vi "dsdll_enumerate_devices.vi"(5 "capture devices ring ref":refnum<vi>, 7 "output devices ring ref":refnum<vi>, 8 "error in":errorcluster, 11 "dsdll instance in":T2={"dsdll path"=path "E:/LVprog/DirectSoundDLL/dsdll.dll", "dsdll handle"=[], "output devices"=[], "capture devices"=[]}) -> (0 "error out":errorcluster, 1 "capture device list":T1[](array[typedef]), 2 "output device list":T1[](array[typedef]), 3 "dsdll instance out":T2)   [LabVIEW 2020, in "dsdll.lvlib"]
doc: "Call this to enumerate output and capture devices. Must be called before opening the audio devices.\n\nThe VI returns lists of output and capture devices and optionally it fills ring buffers with the names of the found devices.\n\nIMPORTANT: The lists of the enumerated devices are also stored in the DSDLL instance handle so don't discard it because it will be later used to open the devices!"
uses:
  dsdll.lvlib
  dsdll_instance.ctl
  dsdll_device_record.ctl
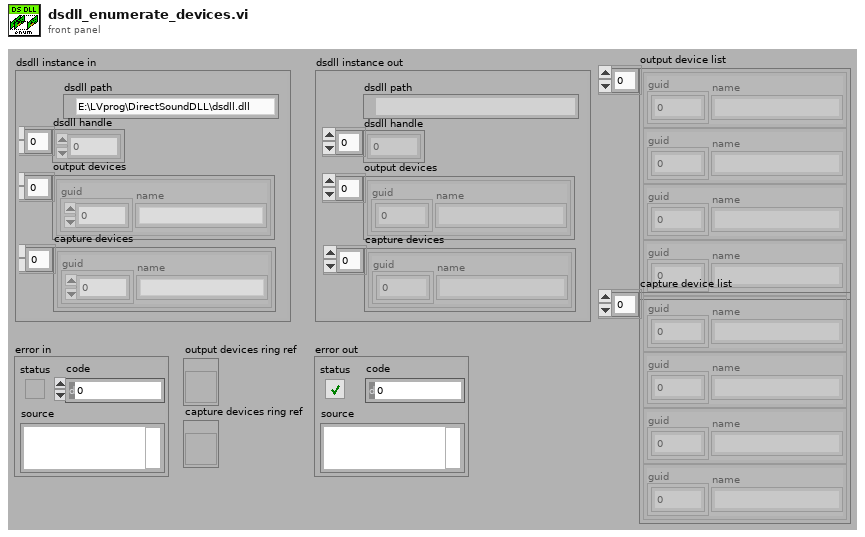
[diagram p1: front panel]
types:
  T1 = typedef "dsdll.lvlib/dsdll_device_record.ctl" = cluster{"guid":u8[], "name":string}
  T2 = typedef "dsdll.lvlib/dsdll_instance.ctl" = cluster{"dsdll path":path, "dsdll handle":u8[], "output devices":T1[], "capture devices":T1[]}
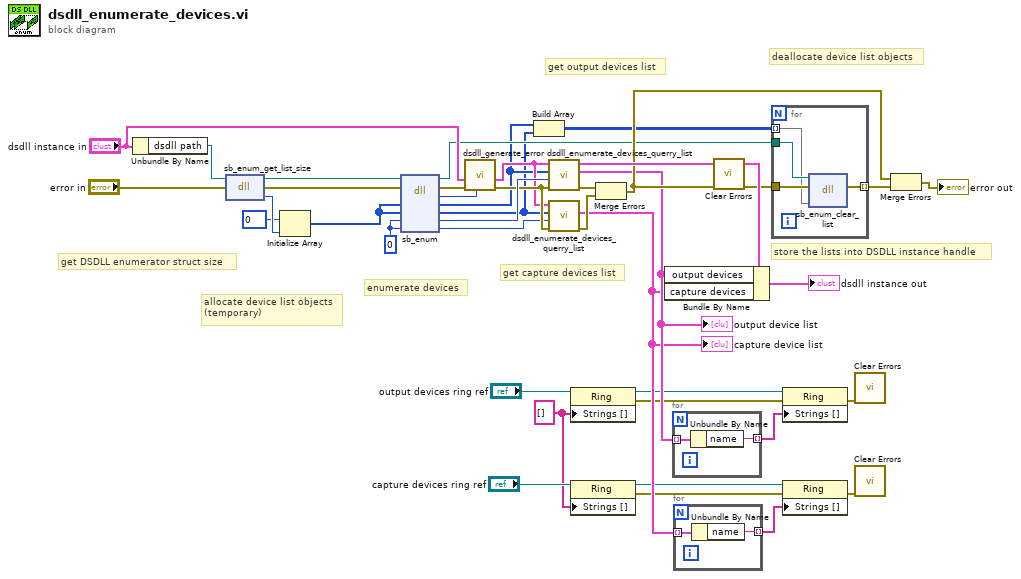
[diagram p0: block diagram]
diagram:
  w1 = string[] [] ("Strings []")
  w31 = 0
  # "deallocate device list objects"
  # "allocate device list objects\n(temporary)"
  # "store the lists into DSDLL instance handle"
  # "get capture devices list"
  # "get output devices list"
  # "enumerate devices"
  # "get DSDLL enumerator struct size"
  n1 = Unbundle By Name("dsdll instance in") -> ("dsdll path"=w39:path)
  n2 = dll-call lib="dsdll.dll" fn="sb_enum_get_list_size" ("sb_get_handle_size()")(path in=w39, error in="error in") -> (path out=w34:path, error out=w38:errorcluster, "size [B]"=w37:u32)  [unwired: 1 in]
  n3 = Initialize Array(u8 0, w37) -> (w30:u8[])
  n4 = dll-call lib="dsdll.dll" fn="sb_enum" ("sb_get_handle_size()")(path in=w34, error in=w38, "output"=w30, "input"=w30, "out_n"=w31, "inp_n"=w31) -> (path out=w18:path, error out=w35:errorcluster, "error"=w32:i32, "output"=w17:u8[], "input"=w16:u8[], "out_n"=w27:i32, "inp_n"=w24:i32)  [unwired: 1 in]
  n5 = call "dsdll_generate_error.vi"("error code"=w32, "error in"=w35, "dsdll instance in"="dsdll instance in") -> ("error out"=w26:errorcluster, "dsdll instance out"=w25:T2)  [unwired: 6 in, 1 out]
  n6 = Build Array(w17, w16) -> (w15:u8[][])
  n7 = call "dsdll_enumerate_devices_querry_list.vi"("error in"=w26, "device count"=w27, "device list object"=w17, "dsdll instance in"=w25) -> ("error out"=w23:errorcluster, "device list"=w13:T1[], "dsdll instance out"=w29:T2)  [unwired: 5 in]
  "output device list" <- w13
  n8 = call "dsdll_enumerate_devices_querry_list.vi"("error in"=w26, "device count"=w24, "device list object"=w16, "dsdll instance in"=w25) -> ("error out"=w22:errorcluster, "device list"=w11:T1[])  [unwired: 5 in, 1 out]
  "capture device list" <- w11
  n9 = property class="Ring"(reference="output devices ring ref", "Strings []"=w1) -> (reference out=w6:refnum<vi>, error out=w5:errorcluster)  [unwired: 1 in]
  n10 = property class="Ring"(reference="capture devices ring ref", "Strings []"=w1) -> (reference out=w3:refnum<vi>, error out=w4:errorcluster)  [unwired: 1 in]
  n11 = Merge Errors(w23, w22) -> (w19:errorcluster)
  n12 = Bundle By Name(cluster=w29, "output devices"=w13, "capture devices"=w11) -> (→"dsdll instance out":T2)
  n13 = for {
    tunnel: w13 -> [w42] mode=indexing
    tunnel: [w41] -> w12 mode=indexing
    n14 = Unbundle By Name(w42) -> ("name"=w41:string)
  }
  n15 = for {
    tunnel: w11 -> [w44] mode=indexing
    tunnel: [w43] -> w10 mode=indexing
    n16 = Unbundle By Name(w44) -> ("name"=w43:string)
  }
  n17 = call <vilib>:"Clear Errors.vi"("error in (no error)"=w19) -> ("error out"=w21:errorcluster)  [unwired: 5 in, 1 out]
  n18 = for {
    tunnel: w21 -> [w48]
    tunnel: [w47] -> w20 mode=indexing
    tunnel: w18 -> [w46]
    tunnel: w15 -> [w45] mode=indexing
    n19 = dll-call lib="dsdll.dll" fn="sb_enum_clear_list" ("sb_get_handle_size()")(path in=w46, error in=w48, "dev_list"=w45) -> (error out=w47:errorcluster)  [unwired: 3 in, 1 out]
  }
  n20 = property class="Ring"(reference=w6, error in=w5, "Strings []"=w12) -> (error out=w9:errorcluster)  [unwired: 1 out]
  n21 = property class="Ring"(reference=w3, error in=w4, "Strings []"=w10) -> (error out=w8:errorcluster)  [unwired: 1 out]
  n22 = call <vilib>:"Clear Errors.vi"("error in (no error)"=w9) -> ()  [unwired: 5 in, 2 out]
  n23 = call <vilib>:"Clear Errors.vi"("error in (no error)"=w8) -> ()  [unwired: 5 in, 2 out]
  n24 = Merge Errors(w19, w20) -> (→"error out":errorcluster)
